vi "Create Transfer Configuration.vi"(6 "settings":T1, 7 "base transfer name (transfer)":string="transfer", 8 "non-random type (DBL)":T2=enum."DBL", 9 "random types? (F)":bool, 11 "channel count":i32) -> (3 "Transfers":T3)   [LabVIEW 2017]
uses:
  Built/Windows/Engine/DSF.Engine.lvlibp/DSF Configuration API/1.0.0/Public/Controls/DSF Engine Transfer Configuration.ctl
  Built/Windows/Engine/DSF.Engine.lvlibp/DSF Configuration API/1.0.0/Public/Controls/DSF Byte Order.ctl
  Built/Windows/Engine/DSF.Engine.lvlibp/DSF Configuration API/1.0.0/Public/Controls/DSF Engine Channel Configuration.ctl
  Built/Windows/Engine/DSF.Engine.lvlibp/DSF Configuration API/1.0.0/Public/Controls/DSF Data Type.ctl
  Built/Windows/Engine/DSF.Engine.lvlibp/DSF Configuration API/1.0.0/Public/Controls/DSF Settings Info.ctl
  Built/Windows/Engine/DSF.Engine.lvlibp/DSF Configuration API/1.0.0/DSF Configuration API.lvlib
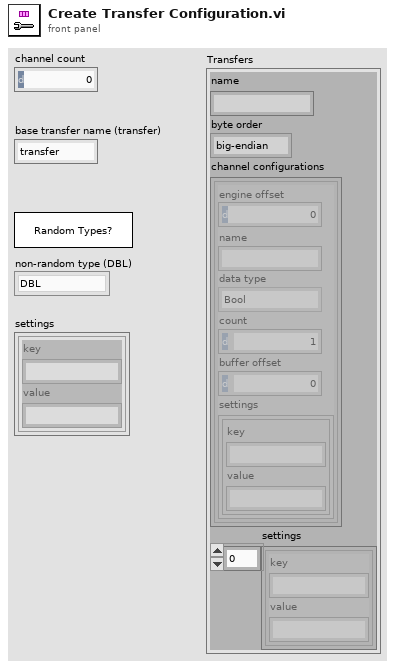
[diagram p1: front panel]
types:
  T1 = typedef "DSF.Engine.lvlibp/DSF Configuration API.lvlib/DSF Settings Info.ctl" = cluster{"key":string, "value":string}[]
  T2 = typedef "DSF.Engine.lvlibp/DSF Configuration API.lvlib/DSF Data Type.ctl" = enum8{"Bool", "SGL", "DBL", "I8", "I16", "I32", "I64", "U8", "U16", "U32", "U64"}
  T3 = typedef "DSF.Engine.lvlibp/DSF Configuration API.lvlib/DSF Engine Transfer Configuration.ctl" = cluster{"name":string, "byte order":T4, "channel configurations":T5[], "settings":T1}
  T4 = typedef "DSF.Engine.lvlibp/DSF Configuration API.lvlib/DSF Byte Order.ctl" = enum8{"big-endian", "little-endian"}
  T5 = typedef "DSF.Engine.lvlibp/DSF Configuration API.lvlib/DSF Engine Channel Configuration.ctl" = cluster{"engine offset":u64, "name":string, "data type":T2, "count":u64, "buffer offset":u64, "settings":T1}
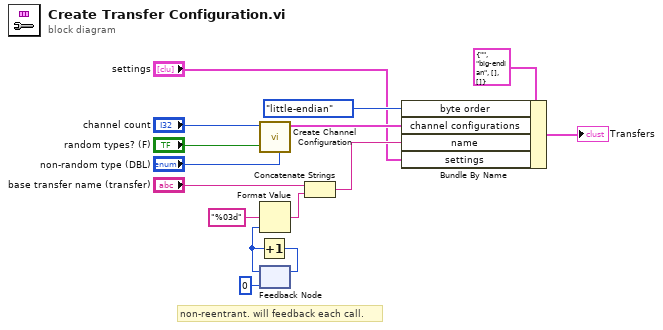
[diagram p0: block diagram]
diagram:
  # "non-reentrant. will feedback each call."
  n1 = call "Create Channel Configuration.vi"("non-random type (DBL)"="non-random type (DBL)", "random types? (F)"="random types? (F)", "channel count"="channel count") -> ("channel configurations"=w4:T5[])  [unwired: 7 in, 1 out]
  n2 = feedback #1(0) -> (w11:i32)
  n3 = Increment(x=w11) -> (x+1=w12:i32)
  n4 = Format Value(format string="%03d", value (0)=w11) -> (output string=w8:string)  [unwired: 1 in]
  n5 = feedback-in #1(w12) -> ()
  n6 = Concatenate Strings("base transfer name (transfer)", w8) -> (w7:string)
  n7 = Bundle By Name(cluster=T3 {"name"="", "byte order"=enum."big-endian", "channel configurations"=[], "settings"=[]} ("Transfers"), "byte order"=DSF_Byte_Order."little-endian", "channel configurations"=w4, "name"=w7, "settings"="settings") -> (→"Transfers":T3)
